vi "Voltage - Finite Input Data Acquisition.vi"(10 "Logging Mode":i32, 11 "TDMS File Path":path) -> (2 "data":waveform(dbl)[](array[waveform]))   [LabVIEW 2017]
uses:
  <vilib>/Utility/error.llb/DialogType.ctl
  <vilib>/DAQmx/read.llb/DAQmx Read (Analog 1D Wfm NChan NSamp).vi
  <vilib>/DAQmx/create/channels.llb/DAQmx Create Channel (AI-Voltage-Basic).vi
  <vilib>/DAQmx/configure/timing.llb/DAQmx Timing (Sample Clock).vi
  <vilib>/DAQmx/configure/task.llb/DAQmx Configure Logging (TDMS).vi
  <vilib>/DAQmx/configure/trigger.llb/DAQmx Start Trigger (Digital Edge).vi
  <vilib>/DAQmx/configure/trigger.llb/DAQmx Start Trigger (Analog Edge).vi
  <vilib>/DAQmx/configure/trigger.llb/DAQmx Reference Trigger (Digital Edge).vi
  <vilib>/DAQmx/configure/trigger.llb/DAQmx Reference Trigger (Analog Edge).vi
  <vilib>/DAQmx/miscellaneous.llb/DAQmx Fill In Error Info.vi
  <resource>/objmgr/daqmx.rc
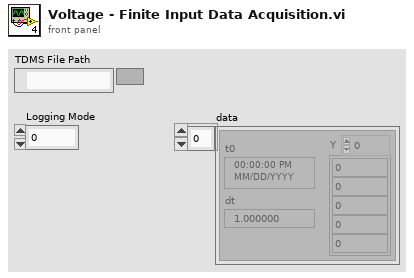
[diagram p1: front panel]
types:
  T1 = enum32{"No Trigger", "Digital Start", "Digital Pause", "Digital Reference", "Analog Start", "Analog Pause", "Analog Reference"}
  T2 = typedef "DialogType.ctl" = u16
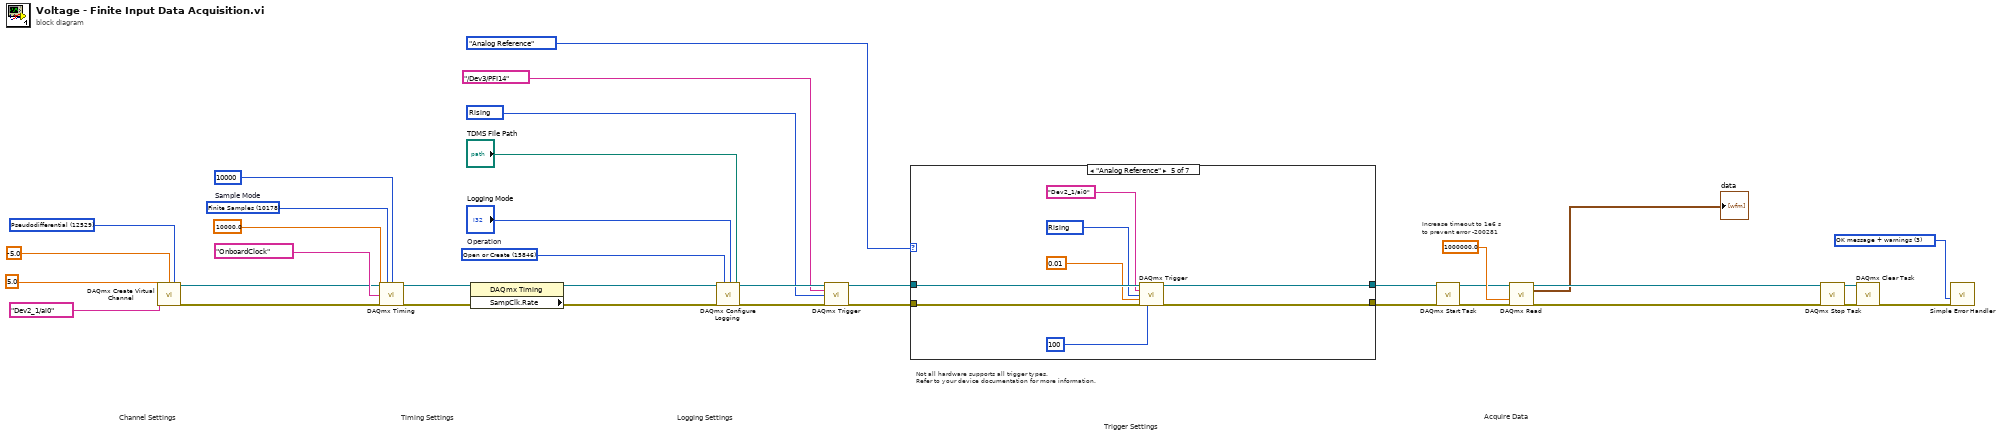
[diagram p0: block diagram]
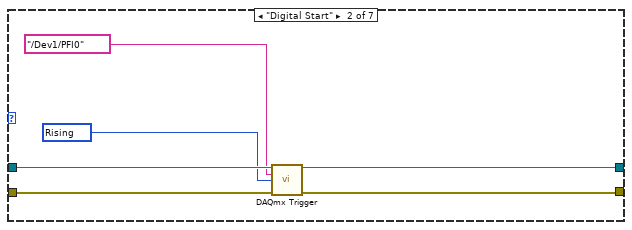
[diagram p3: hidden frame]
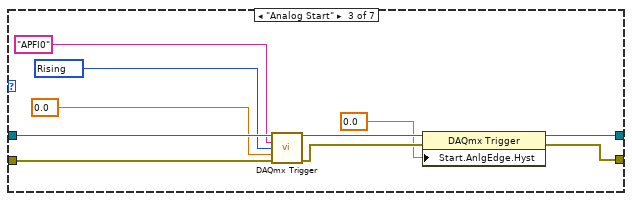
[diagram p4: hidden frame]
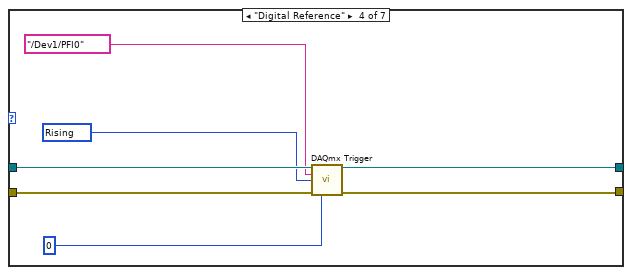
[diagram p5: hidden frame]
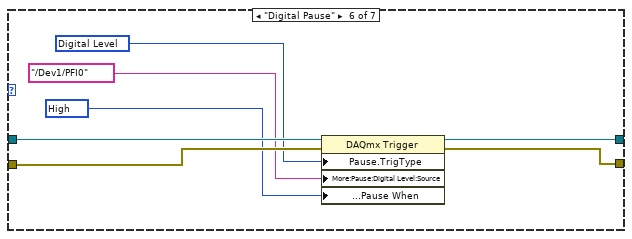
[diagram p6: hidden frame]
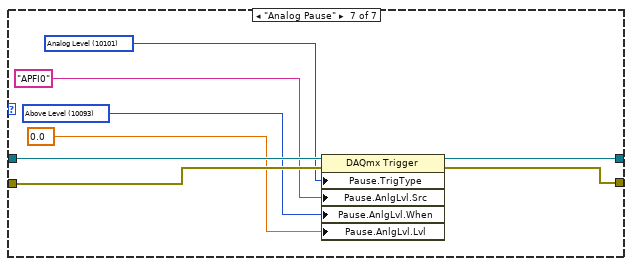
[diagram p7: hidden frame]
diagram:
  w1 = 10280 items=["Rising"=10280, "Falling"=10171] ("edge")
  w21 = 12529 items=["default"=-1, "RSE"=10083, "NRSE"=10078, "Differential"=10106, "Pseudodifferential"=12529] ("Terminal Configuration")
  w33 = T2 3 items=["no dialog", "OK message", "continue or stop message", "OK message + warnings", "continue/stop + warnings"] ("type of dialog (OK msg:1)")
  w15 = 15846 items=["Open"=10437, "Open or Create"=15846, "Create or Replace"=15847, "Create"=15848]  # Operation
  w10 = 10178 items=["Finite Samples"=10178, "Continuous Samples"=10123, "Hardware Timed Single Point"=12522]  # Sample Mode
  # "Increase timeout to 1e6 s\nto prevent error -200281"
  # "Not all hardware supports all trigger types.\nRefer to your device documentation for more information."
  # "Trigger Settings"
  # "Acquire Data"
  # "Timing Settings"
  # "Channel Settings"
  # "Logging Settings"
  n1 = call-poly <vilib>:"DAQmx Create Virtual Channel.vi"("maximum value"=5.0 ("Max Voltage"), "minimum value"=-5.0 ("Min Voltage"), "input terminal configuration"=w21, "physical channels"=tag "Dev2_1/ai0" ("Physical Channel")) -> ("task out"=w12:refnum<k21>, "error out"=w11:errorcluster)  [unwired: 10 in]
  n2 = call-poly <vilib>:"DAQmx Timing.vi"("task/channels in"=w12, "sample mode"=w10, "samples per channel"=10000 ("Number of Samples"), "rate"=10000.0 ("Sample Rate"), "source"=tag "OnboardClock" ("Sample Clock Source"), "error in"=w11) -> ("task out"=w8:refnum<k21>, "error out"=w9:errorcluster)  [unwired: 8 in]
  n3 = property class="DAQmx Timing" props=["SampClk.Rate"](reference=w8, error in=w9) -> (reference out=w13:refnum<k21>, error out=w14:errorcluster)  [unwired: 1 out]
  n4 = call-poly <vilib>:"DAQmx Configure Logging.vi"("task/channels in"=w13, "operation"=w15, "file path"="TDMS File Path", "logging mode"="Logging Mode", "error in"=w14) -> ("task out"=w6:refnum<k21>, "error out"=w4:errorcluster)  [unwired: 9 in]
  n5 = call-poly <vilib>:"DAQmx Trigger.vi"("task/channels in"=w6, "source"=tag "/Dev3/PFI14", "edge"=w1, "error in"=w4) -> ("task out"=w5:refnum<k21>, "error out"=w3:errorcluster)  [unwired: 10 in]
  n6 = case shown="\"Analog Reference\"" T1."Analog Reference" ("Trigger Type") {
    tunnel: w5 -> [w38 w44 w54 w61 w69 w76 w84]
    tunnel: w3 -> [w37 w43 w53 w60 w68 w73 w81]
    tunnel: [w38 w42 w51 w59 w67 w75 w83] -> w7
    tunnel: [w37 w41 w50 w58 w66 w74 w82] -> w35
    frame "No Trigger", Default {
    }
    frame "Digital Start" {
      w40 = 10280 items=["Rising"=10280, "Falling"=10171] ("Digital Start Trigger Edge")
      n7 = call-poly <vilib>:"DAQmx Trigger.vi"("task/channels in"=w44, "source"=tag "/Dev1/PFI0" ("Digital Start Trigger Source"), "edge"=w40, "error in"=w43) -> ("task out"=w42:refnum<k21>, "error out"=w41:errorcluster)  [unwired: 10 in]
    }
    frame "Analog Start" {
      w52 = 10280 items=["Rising"=10280, "Falling"=10171] ("Analog Start Trigger Slope")
      n8 = call-poly <vilib>:"DAQmx Trigger.vi"("task/channels in"=w54, "source"="APFI0" ("Analog Start Trigger Source"), "slope"=w52, "level"=0.0 ("Analog Start Trigger Level"), "error in"=w53) -> ("task out"=w49:refnum<k21>, "error out"=w48:errorcluster)  [unwired: 9 in]
      n9 = property class="DAQmx Trigger"(reference=w49, error in=w48, "Start.AnlgEdge.Hyst"=0.0 ("Analog Start Trigger Hysteresis")) -> (reference out=w51:refnum<k21>, error out=w50:errorcluster)
    }
    frame "Digital Reference" {
      w55 = 10280 items=["Rising"=10280, "Falling"=10171] ("Digital Reference Trigger Edge")
      n10 = call-poly <vilib>:"DAQmx Trigger.vi"("task/channels in"=w61, "source"=tag "/Dev1/PFI0" ("Digital Reference Trigger Source"), "edge"=w55, "error in"=w60, "pretrigger samples per channel"=u32 0 ("Digital Reference Pretrigger Samples")) -> ("task out"=w59:refnum<k21>, "error out"=w58:errorcluster)  [unwired: 9 in]
    }
    frame "Analog Reference" {
      w64 = 10280 items=["Rising"=10280, "Falling"=10171] ("Analog Reference Trigger Slope")
      n11 = call-poly <vilib>:"DAQmx Trigger.vi"("task/channels in"=w69, "source"="Dev2_1/ai0" ("Analog Reference Trigger Source"), "slope"=w64, "level"=0.01 ("Analog Reference Trigger Level"), "error in"=w68, "pretrigger samples per channel"=u32 100 ("Analog Reference Pretrigger Samples")) -> ("task out"=w67:refnum<k21>, "error out"=w66:errorcluster)  [unwired: 8 in]
    }
    frame "Digital Pause" {
      w70 = 10192 items=["High"=10192, "Low"=10214] ("Digital Pause Trigger Pause When")
      w72 = 10152 items=["Analog Level"=10101, "Analog Window"=10103, "Digital Level"=10152, "Digital Pattern"=10398, "None"=10230] ("Pause.TrigType")
      n12 = property class="DAQmx Trigger"(reference=w76, error in=w73, "Pause.TrigType"=w72, "More:Pause:Digital Level:Source"=tag "/Dev1/PFI0" ("Digital Pause Trigger Source"), "More:Pause:Digital Level:Pause When"=w70) -> (reference out=w75:refnum<k21>, error out=w74:errorcluster)
    }
    frame "Analog Pause" {
      w78 = 10093 items=["Above Level"=10093, "Below Level"=10107] ("Analog Pause Trigger Pause When")
      w80 = 10101 items=["Analog Level"=10101, "Analog Window"=10103, "Digital Level"=10152, "Digital Pattern"=10398, "None"=10230] ("Pause.TrigType")
      n13 = property class="DAQmx Trigger"(reference=w84, error in=w81, "Pause.TrigType"=w80, "Pause.AnlgLvl.Src"="APFI0" ("Analog Pause Trigger Source"), "Pause.AnlgLvl.When"=w78, "Pause.AnlgLvl.Lvl"=0.0 ("Analog Pause Trigger Level")) -> (reference out=w83:refnum<k21>, error out=w82:errorcluster)
    }
  }
  n14 = call <vilib>:"DAQmx Start Task.vi"("task/channels in"=w7, "error in"=w35) -> ("task out"=w16:refnum<k21>, "error out"=w17:errorcluster)  [unwired: 12 in]
  n15 = call-poly <vilib>:"DAQmx Read.vi"("task/channels in"=w16, "timeout"=1000000.0, "error in"=w17) -> ("task out"=w31:refnum<k21>, "data"=→"data":waveform(dbl)[], "error out"=w32:errorcluster)  [unwired: 10 in]
  n16 = call <vilib>:"DAQmx Stop Task.vi"("task/channels in"=w31, "error in"=w32) -> ("task out"=w29:refnum<k21>, "error out"=w30:errorcluster)  [unwired: 12 in]
  n17 = call <vilib>:"DAQmx Clear Task.vi"("task in"=w29, "error in"=w30) -> ("error out"=w18:errorcluster)  [unwired: 13 in]
  n18 = call <vilib>:"Simple Error Handler.vi"("type of dialog (OK msg:1)"=w33, "error in (no error)"=w18) -> ()  [unwired: 3 in, 5 out]
